vi "event_functional_load_interface.vi"(6 "functional":refnum<user-event>, 8 "error in (no error)":errorcluster, 11 "interface":refnum<class "interface.lvclass">) -> (0 "error out":errorcluster)   [LabVIEW 2015, in "functional.lvlib"]
uses:
  functional.lvlib
  example/example_01/functional/public/interface/interface.lvclass
  _controls/event_functional.ctl
  _controls/event_functional_command.ctl
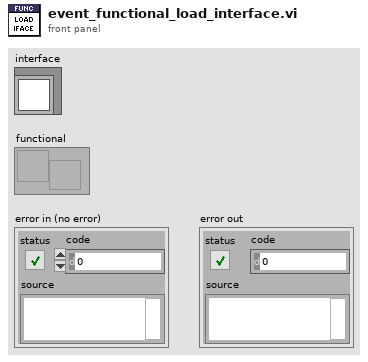
[diagram p1: front panel]
types:
  T1 = typedef "functional.lvlib/event_functional_command.ctl" = enum16{"<command_functional>", "--high-level", "stop", "update_hmi_references", "load_interface", "--functional", "do_it", "<null>"}
  T2 = typedef "functional.lvlib/event_functional.ctl" = cluster{"command":T1, "data":variant}
  T3 = cluster{"queue out":refnum<queue>, "interface":refnum<class "interface.lvclass">}
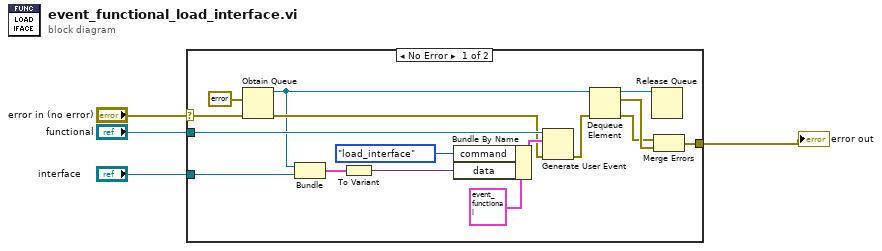
[diagram p0: block diagram]
diagram:
  n1 = case shown="No Error" "error in (no error)" {
    selector: "error in (no error)" -> [w14 w21]
    tunnel: "functional" -> [w16 _]
    tunnel: [w10 w21] -> w2
    tunnel: "interface" -> [w7 _]
    frame No Error {
      n2 = Obtain Queue(element data type=errorcluster {"status"=FALSE, "code"=0, "source"=""} ("error in (no error)"), error in (no error)=w14) -> (queue out=w5:refnum<queue>, error out=w12:errorcluster)  [unwired: 3 in, 1 out]
      n3 = Bundle("queue out"=w5, "interface"=w7) -> (w8:T3)  [unwired: 1 in]
      n4 = To Variant(anything=w8) -> (Variant=w20:variant)
      n5 = Bundle By Name(cluster=T2 {"command"=enum."<command_functional>", "data"=variant} ("event data"), "command"=event_functional_command."load_interface", "data"=w20) -> (w17:T2)
      n6 = Generate User Event(user event=w16, event data cluster=w17, error in=w12) -> (error out=w11:errorcluster)  [unwired: 1 in, 1 out]
      n7 = Dequeue Element(queue=w5, error in (no error)=w11) -> (queue out=w13:refnum<queue>, element=w9:errorcluster, error out=w6:errorcluster)  [unwired: 1 in, 1 out]
      n8 = Release Queue(queue=w13) -> ()  [unwired: 2 in, 3 out]
      n9 = Merge Errors(w6, w9) -> (w10:errorcluster)
    }
    frame Error {
    }
  }
  "error out" <- w2
